vi "SetOverlayPositionAndBounds.vi"(8 "error in (no error)":errorcluster, 10 "item index":i32, 11 "menu in":refnum<class "menu.lvclass">) -> (0 "error out":errorcluster, 3 "menu out":refnum<class "menu.lvclass">)   [LabVIEW 2009, in "menu.lvclass"]
uses:
  menu.lvclass
  menu.lvclass/menu.ctl
  Menu Item/menu item.lvclass
  Overlay/overlay.lvclass
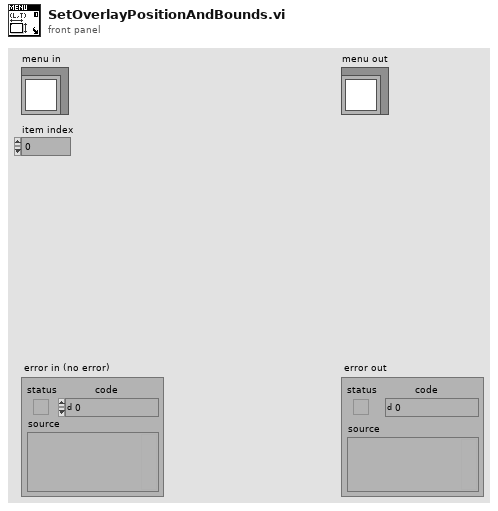
[diagram p1: front panel]
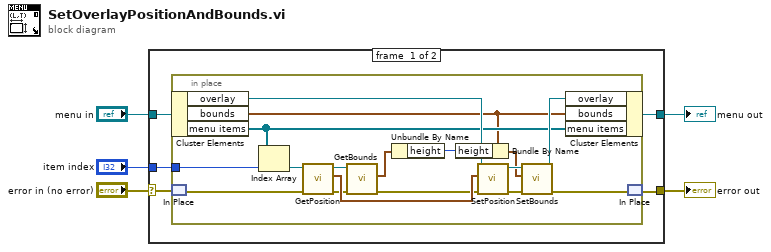
[diagram p0: block diagram]
diagram:
  n1 = case shown="No Error" "error in (no error)" {
    selector: "error in (no error)" -> [w8 w29]
    tunnel: [w7 w29] -> w2
    tunnel: [w9 w28] -> w4
    tunnel: "menu in" -> [w10 w28]
    tunnel: "item index" -> [w6 _]
    frame #0 {
      n2 = in-place {
        in-place-border: w6 -> [w22]
        n3 = in-place-cluster #1(w10) -> ("overlay"=w26:refnum<class "overlay.lvclass">, "bounds"=w21:cluster{"width":u32, "height":u32}, "menu items"=w23:refnum<class "menu item.lvclass">[])
        n4 = in-place-match #2(w8) -> (w25:errorcluster)
        n5 = Index Array(array=w23, index=w22) -> (element=w13:refnum<class "menu item.lvclass">)
        n6 = call-dynamic "GetPosition.vi"("error in (no error)"=w25, "menu item in"=w13) -> ("error out"=w17:errorcluster, "position"=w18:cluster{"left":u32, "top":u32}, "menu item out"=w16:refnum<class "menu item.lvclass">)  [unwired: 7 in]
        n7 = call-dynamic "GetBounds.vi"("error in (no error)"=w17, "menu item in"=w16) -> ("error out"=w12:errorcluster, "bounds"=w19:cluster{"width":u32, "height":u32})  [unwired: 7 in, 1 out]
        n8 = Unbundle By Name(w19) -> ("height"=w20:u32)
        n9 = Bundle By Name(cluster=w21, "height"=w20) -> (w11:cluster{"width":u32, "height":u32})
        n10 = call "SetPosition.vi"("error in (no error)"=w12, "position"=w18, "overlay in"=w26) -> ("error out"=w15:errorcluster, "overlay out"=w14:refnum<class "overlay.lvclass">)  [unwired: 7 in]
        n11 = call "SetBounds.vi"("error in (no error)"=w15, "bounds"=w11, "overlay in"=w14) -> ("error out"=w24:errorcluster, "overlay out"=w27:refnum<class "overlay.lvclass">)  [unwired: 7 in]
        n12 = in-place-cluster #1("overlay"=w27, "bounds"=w21, "menu items"=w23) -> (w9:refnum<class "menu.lvclass">)
        n13 = in-place-match #2(w24) -> (w7:errorcluster)
      }
    }
    frame #1 {
    }
  }
  "menu out" <- w4
  "error out" <- w2
